vi "BinaryOutput.vi"(8 "Current Threshold":dbl=1000.0 format="%#_13g", 11 "Current Level of Output Pins 2":dbl[](array[numeric])) -> (2 "Actual Binary\nOutput":bool[](array[boolean]), 3 "Current Level of Output Pins":dbl[](array[numeric]))   [LabVIEW 2018]
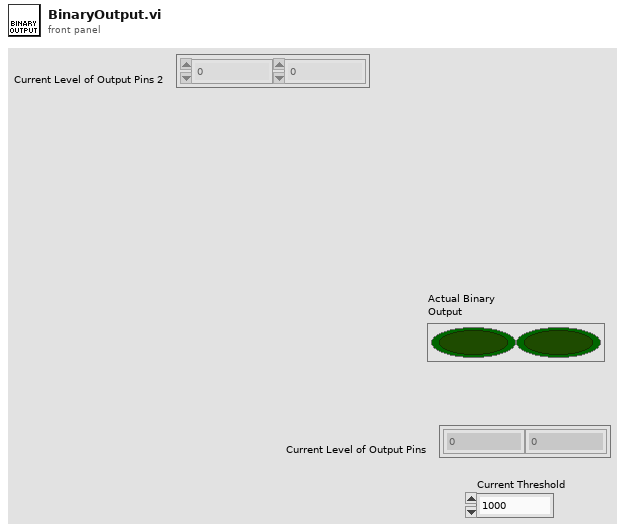
[diagram p1: front panel]
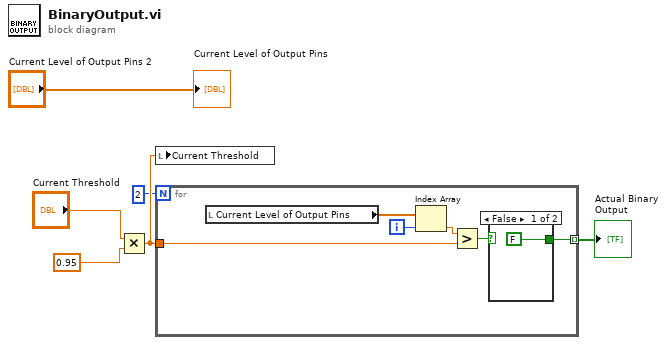
[diagram p0: block diagram]
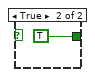
[diagram p2: hidden frame]
diagram:
  n1 = Multiply(x="Current Threshold", y=0.95) -> (x*y=w3:dbl)
  n2 = local write "Current Threshold"(w3) -> ()
  n3 = for {
    N: 2 -> [_]
    tunnel: w3 -> [w9]
    tunnel: [w7] -> w6 mode=indexing
    i -> [w8]
    n4 = local read "Current Level of Output Pins"() -> (w11:dbl[])
    n5 = Index Array(array=w11, index=w8) -> (element=w10:dbl)
    n6 = Greater?(x=w10, y=w9) -> (0:w12:bool)
    n7 = case shown="False" w12 {
      tunnel: [FALSE TRUE] -> w7
      frame False {
      }
      frame True {
      }
    }
  }
  "Actual Binary\nOutput" <- w6
  "Current Level of Output Pins" <- "Current Level of Output Pins 2"
